vi "LHF.DB.Mongo.Bson.FromVariant.vi"(0 "Variant":variant, 5 "error IO":errorcluster) -> (14 "BsonValue":refnum<k24>, 19 "error IO 2":errorcluster)   [LabVIEW 2013, in "LHF.DB.Mongo.lvclass"]
uses:
  LHF.DB.Mongo.lvclass
  C:/Users/Ricardo/Desktop/Projetos/LabVIEW-MongoDB/src/Driver/MongoDB.Bson.dll
  Driver/MongoDB.Bson.dll
  <vilib>/Utility/VariantDataType/VariantType.lvlib
panel:
  in  "Treatment of Infinity/NaN":T1(ring)
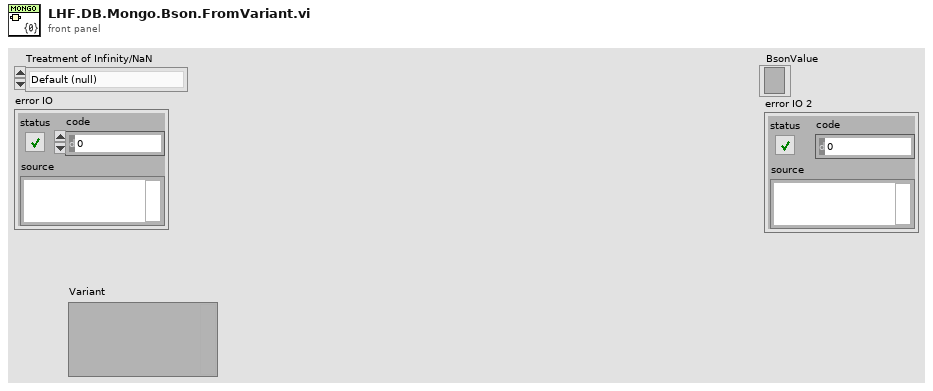
[diagram p1: front panel]
types:
  T1 = enum16{"Default (null)", "Extended", "LabVIEW extensions"}
  T2 = typedef "VariantType.lvlib/Type.ctl" = enum8{"Invalid Type", "Void", "I8", "I16", "I32", "I64", "U8", "U16", "U32", "U64", "Single Float", "Double Float", "Extended Float", "Single Complex", "Double Complex", "Extended Complex", "Enum U8", "Enum U16", "Enum U32", "Enum U64", "Single Float With Unit", "Double Float With Unit", "Extended Float With Unit", "Single Complex with Unit", "Double Complex with Unit", "Extended Complex with Unit", "Boolean", "String", "Path", "Picture", "Tag", "Array", "Cluster", "Variant", "LV Variant", "Waveform", "Timestamp", "Digital Waveform", "Digital Data", "ExpressData", "Refnum", "External Data", "VI", "Poly VI", "LabVIEW Class Instance", "Fixed Point"}
  T3 = typedef "LHF.DB.Mongo.lvclass/LHF.DB.Mongo.Typedef.VariantData.ctl" = cluster{"Type Enum":T2, "Name":string, "Variant":variant}
  T4 = typedef "VariantType.lvlib/RefnumType.ctl" = enum16{"NotARefnum", "UnknownRefnum", "Generic", "Datalog", "ByteStream", "Device", "Occurence", "TCPNetConnection", "Auto", "Menu", "Imaq", "Hardware", "DataSocket", "Visa", "IVI", "UDPNetConnection", "Notifier", "Queue", "Irda", "EventReg", "DotNet", "UserEvent", "Callback", "UNUSED_EMPTY_POSITION", "BlueToothNetConnection", "LVObjApp", "LVObjVI", "LVObjUnknown", "GenericClass", "UserDefinedRefnumTag", "DataValue", "RT FIFO", "TDMS File"}
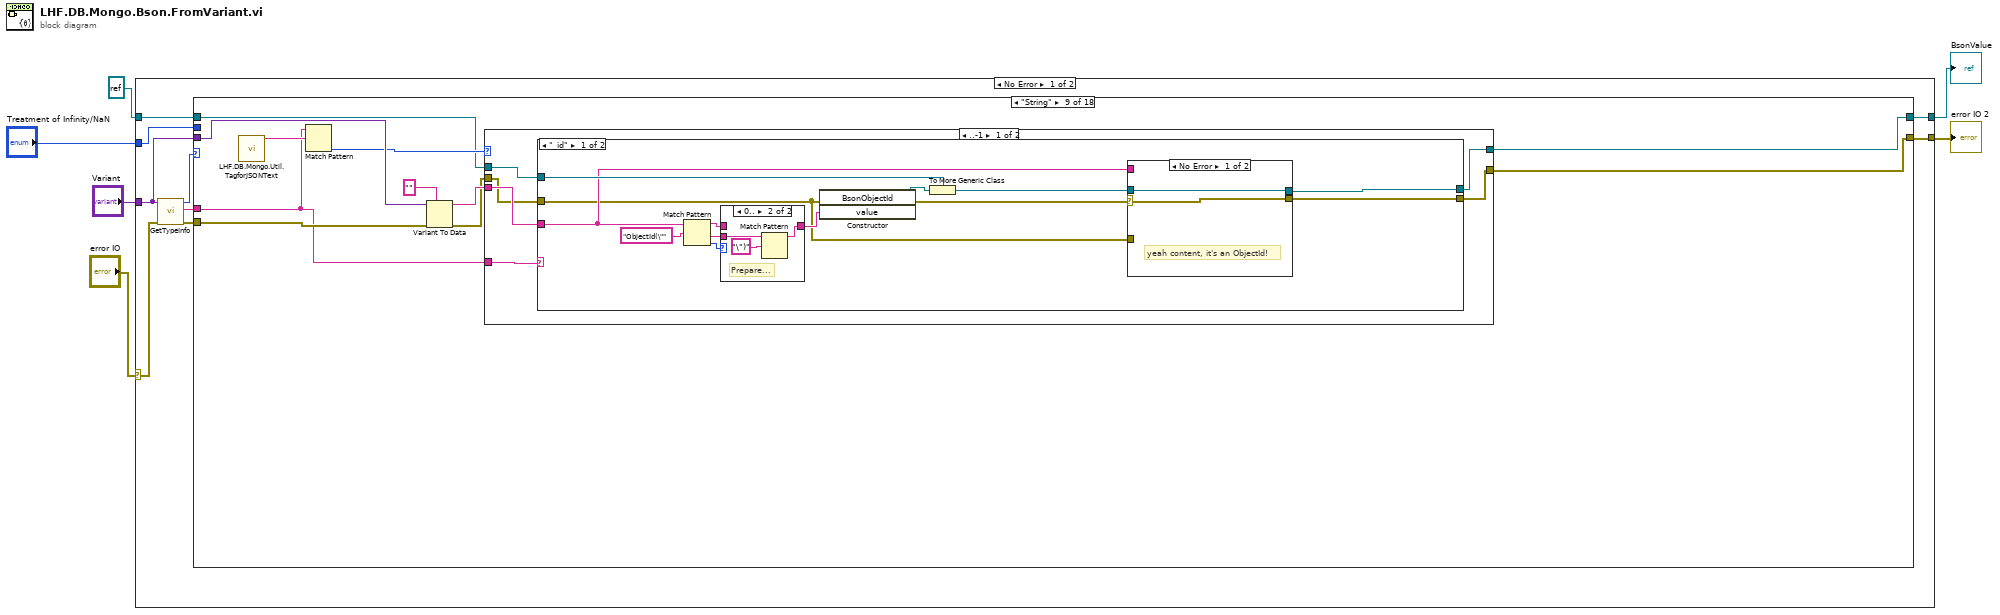
[diagram p0: block diagram]
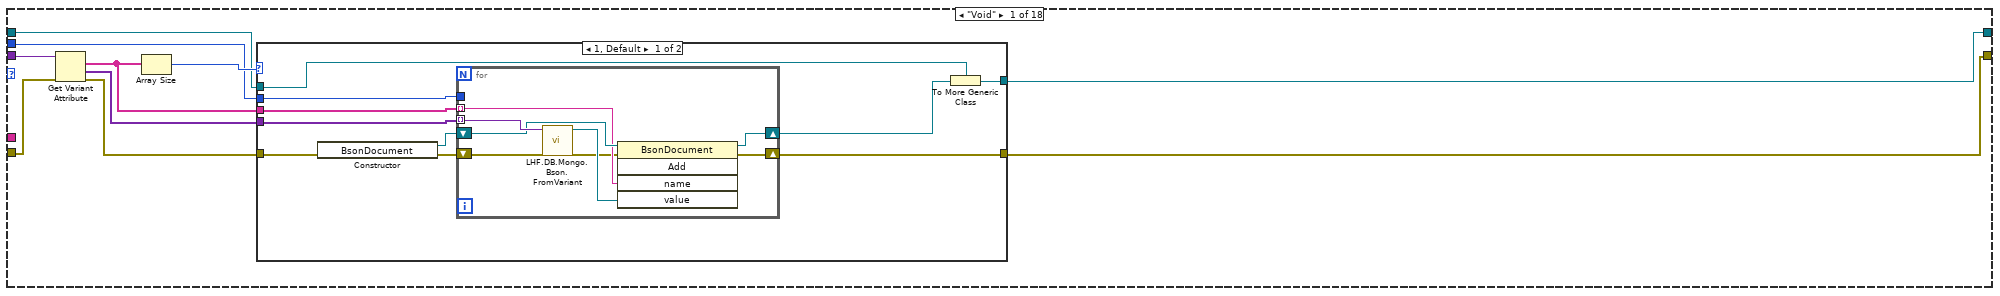
[diagram p2: hidden frame]
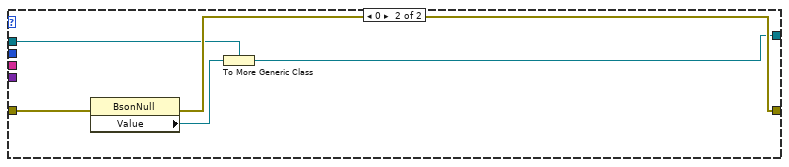
[diagram p3: hidden frame]
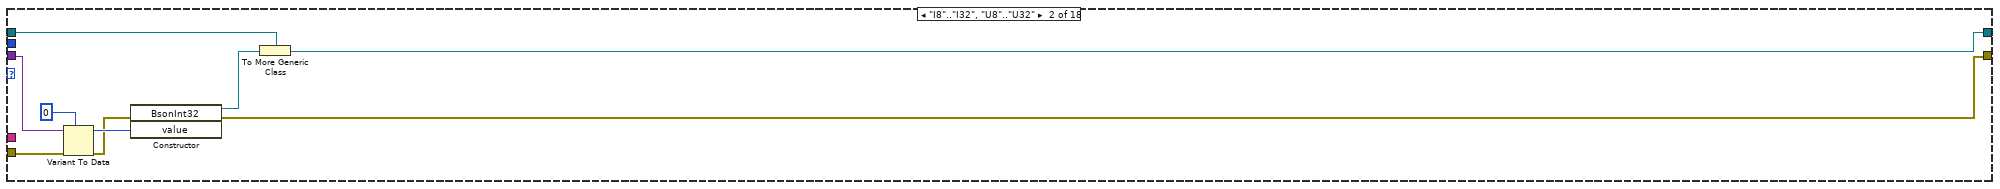
[diagram p4: hidden frame]
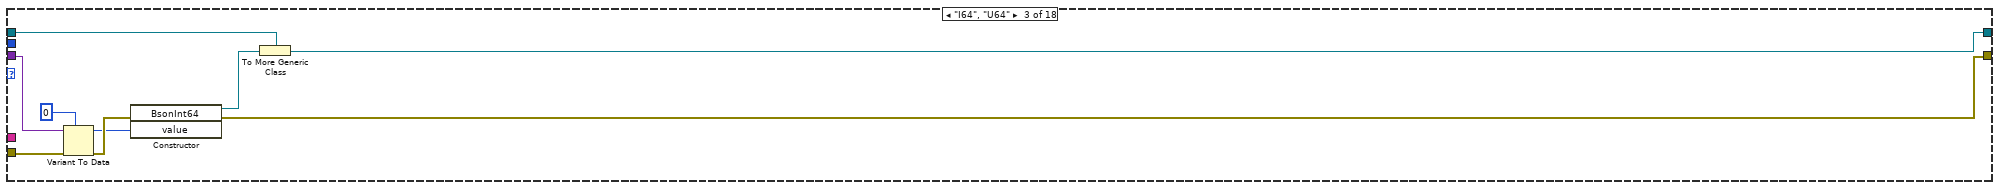
[diagram p5: hidden frame]
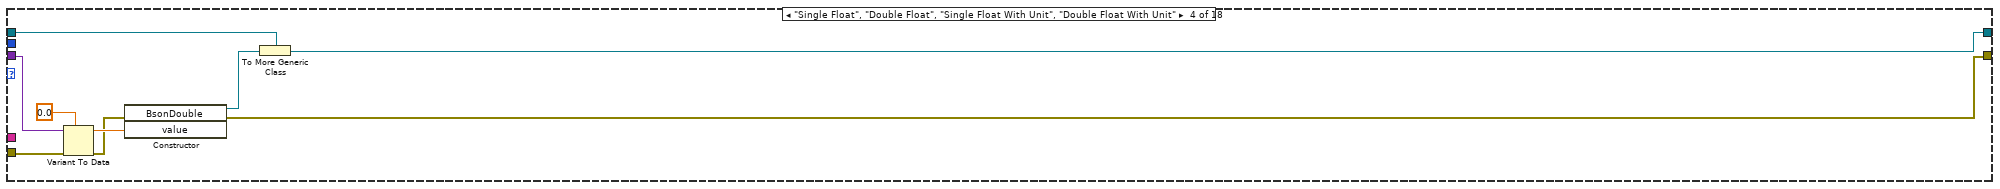
[diagram p6: hidden frame]
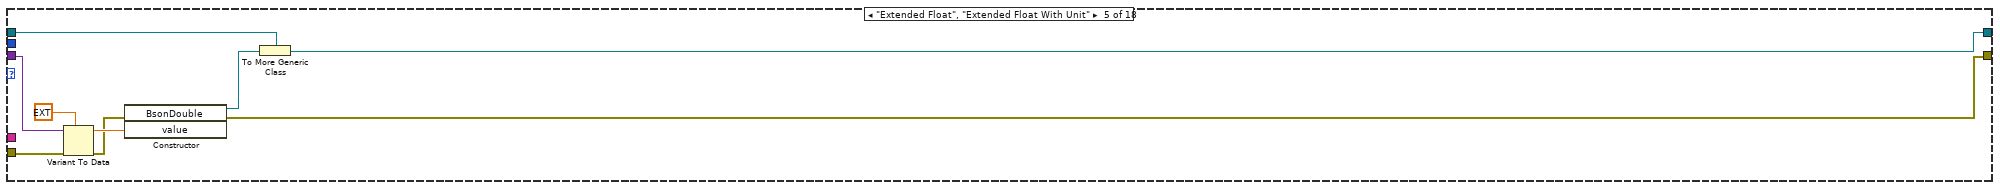
[diagram p7: hidden frame]
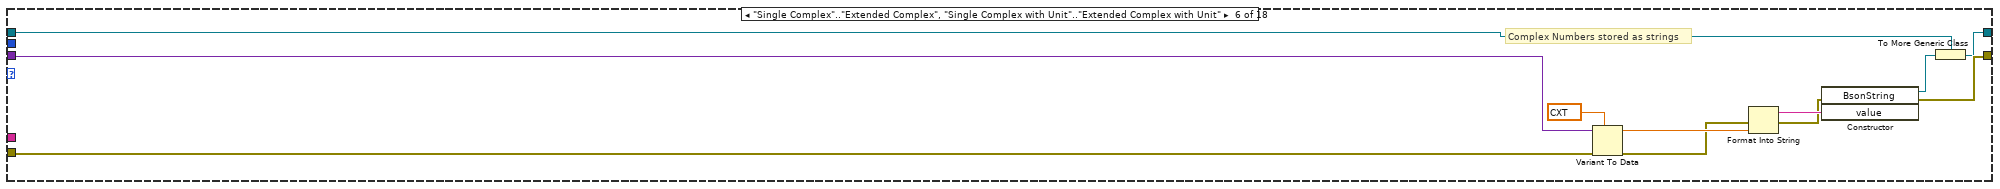
[diagram p8: hidden frame]
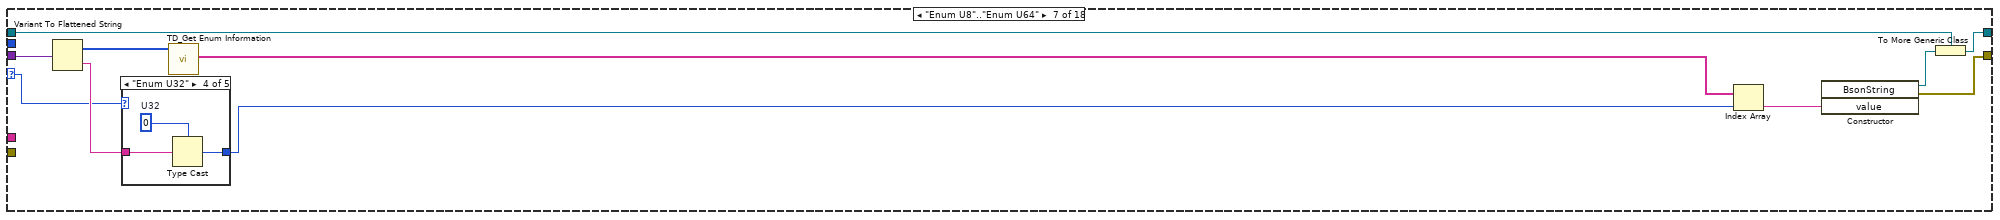
[diagram p9: hidden frame]
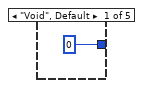
[diagram p10: hidden frame]
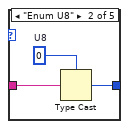
[diagram p11: hidden frame]
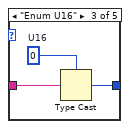
[diagram p12: hidden frame]
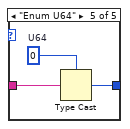
[diagram p13: hidden frame]
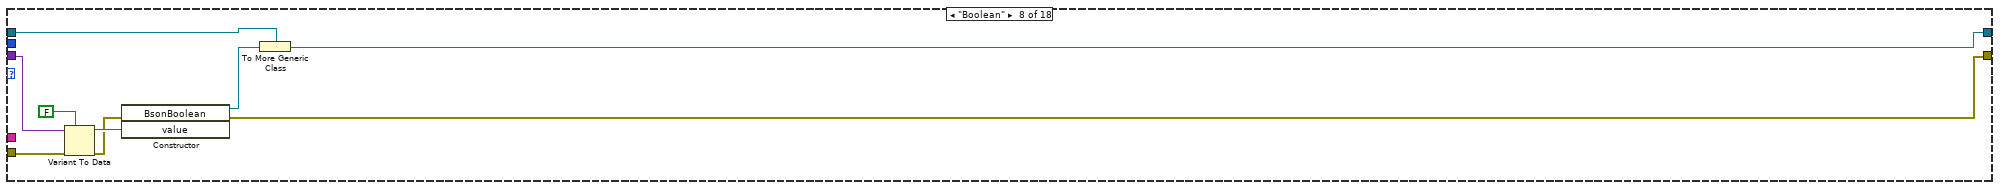
[diagram p14: hidden frame]
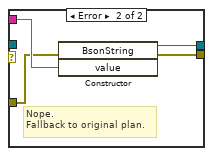
[diagram p15: hidden frame]
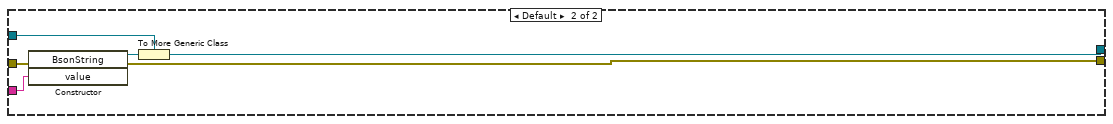
[diagram p17: hidden frame]
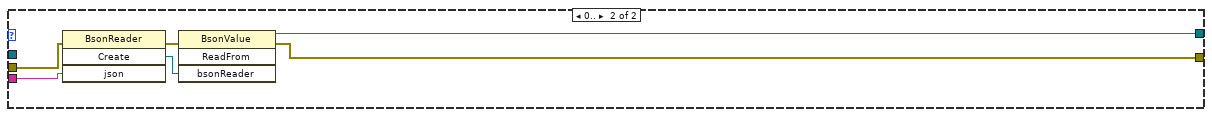
[diagram p18: hidden frame]
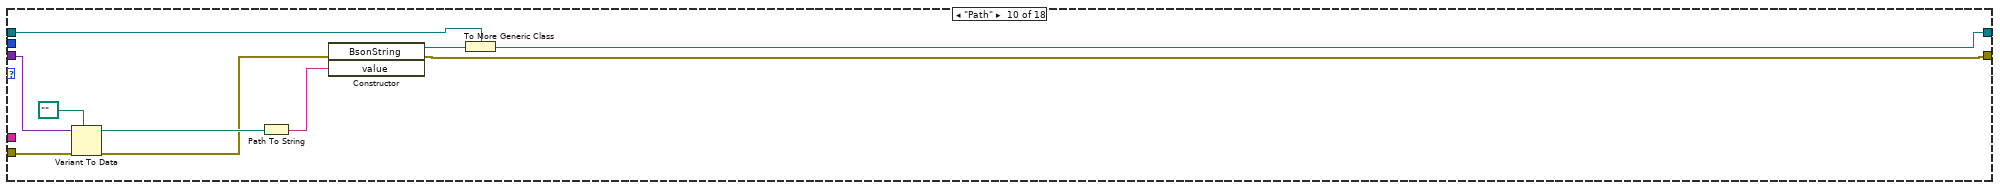
[diagram p19: hidden frame]
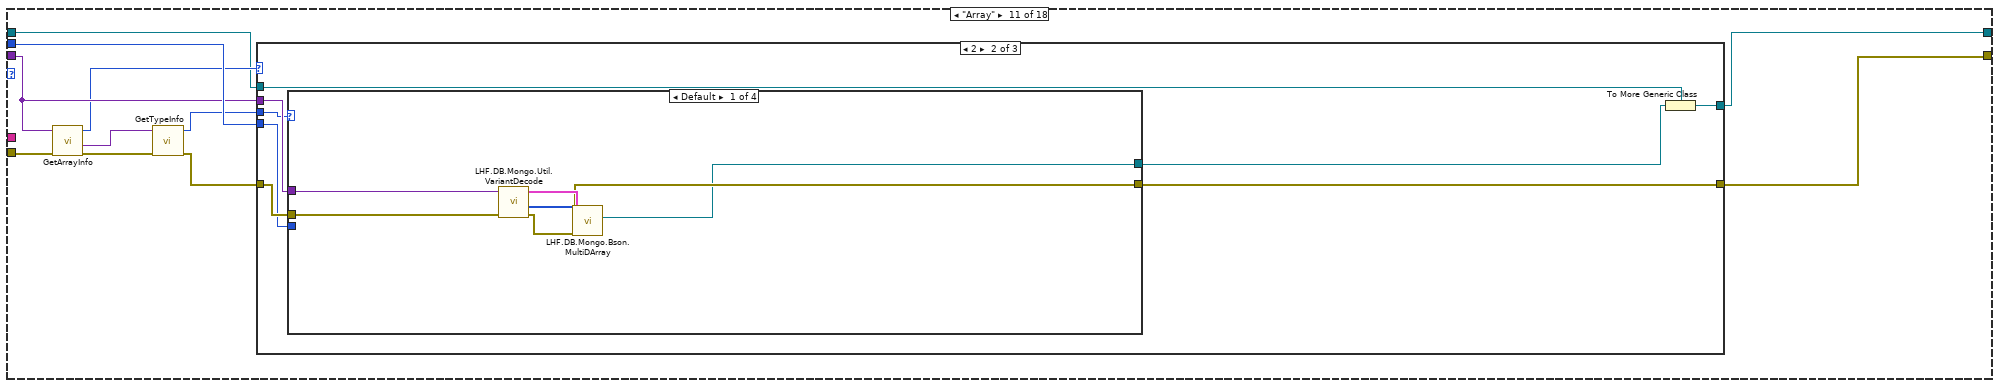
[diagram p20: hidden frame]
diagram:
  n1 = case shown="No Error" "error IO" {
    selector: "error IO" -> [w13 w488]
    tunnel: [w15 w488] -> w1
    tunnel: "Variant" -> [w14 _]
    tunnel: "Treatment of Infinity/NaN" -> [w9 _]
    tunnel: [w8 w487] -> w3
    tunnel: refnum<k24> refnum ("new reference") -> [w7 w487]
    frame No Error {
      n2 = call <vilib>:"GetTypeInfo.vi"("error in (no error)"=w13, "Variant"=w14) -> ("error out"=w12:errorcluster, "Name"=w10:string, "Type Enum"=w11:T2)  [unwired: 5 in, 2 out]
      n3 = case shown="\"String\"" w11 {
        selector: w11 -> [_ _ _ _ _ _ w101 _ _ _ _ _ _ _ _ _ _ _]
        tunnel: w14 -> [w24 w57 w66 w75 w84 w95 w102 w128 w139 w190 w199 w403 w423 w433 w442 w450 w479 w486]
        tunnel: [w25 w52 w63 w68 w79 w88 w98 w122 w135 w184 w201 w405 w419 w428 w437 w444 w471 w482] -> w15
        tunnel: w12 -> [w19 w55 w64 w73 w82 w94 _ w126 w134 w188 w198 w401 w422 w432 w440 w449 w478 w483]
        tunnel: w10 -> [_ _ _ _ _ _ _ _ w129 _ _ _ _ _ _ _ _ _]
        tunnel: w9 -> [w18 _ _ _ _ _ _ _ _ _ w200 w400 _ _ _ _ _ _]
        tunnel: [w16 w49 w58 w67 w76 w85 w96 w120 w131 w181 w191 w396 w416 w425 w435 w443 w469 w480] -> w8
        tunnel: w7 -> [w17 w50 w59 w70 w77 w86 w97 w123 w132 w182 w192 w397 w418 w427 w434 w446 w470 w481]
        frame "Void" {
          n4 = Get Variant Attribute(Variant=w24, error in=w19) -> (names=w22:string[], values=w21:variant[], error out=w20:errorcluster)  [unwired: 2 in, 1 out]
          n5 = Array Size(array=w22) -> (size(s)=w23:i32)
          n6 = case shown="1, Default" w23 {
            tunnel: [w33 w48] -> w25
            tunnel: w22 -> [w34 _]
            tunnel: w21 -> [w35 _]
            tunnel: w20 -> [w26 w47]
            tunnel: w18 -> [w32 _]
            tunnel: w17 -> [w28 w45]
            tunnel: [w29 w44] -> w16
            frame 1, Default {
              n7 = constructor class="BsonDocument"(error in=w26) -> (reference out=w31:refnum<k24>, error out=w27:errorcluster)  [unwired: 2 in, 1 out]
              n8 = for {
                tunnel: w35 -> [w43] mode=indexing
                shift-right: [w36] -> w33
                shift-left: w27 -> [w37]
                tunnel: w34 -> [w40] mode=indexing
                shift-right: [w41] -> w30
                shift-left: w31 -> [w42]
                tunnel: w32 -> [_]
                n9 = call "LHF.DB.Mongo.Bson.FromVariant.vi"("Variant"=w43, "error IO"=w37) -> ("BsonValue"=w39:refnum<k24>, "error IO 2"=w38:errorcluster)  [unwired: 16 in]
                n10 = invoke class="BsonDocument" method="Add"(reference=w42, error in=w38, "name"=w40, "value"=w39) -> (reference out=w41:refnum<k24>, error out=w36:errorcluster)  [unwired: 1 in, 3 out]
              }
              n11 = To More Generic Class(target class=w28, reference=w30) -> (generic class reference=w29:refnum<k24>)
            }
            frame 0 {
              n12 = property class="BsonNull"(error in=w47) -> (error out=w48:errorcluster, "Value"=w46:refnum<k24>)  [unwired: 1 in, 1 out]
              n13 = To More Generic Class(target class=w45, reference=w46) -> (generic class reference=w44:refnum<k24>)
            }
          }
        }
        frame "I8".."I32", "U8".."U32" {
          n14 = Variant To Data(error in=w55, type=0, Variant=w57) -> (data=w54:i32, error out=w53:errorcluster)
          n15 = constructor class="BsonInt32"(error in=w53, "value"=w54) -> (reference out=w51:refnum<k24>, error out=w52:errorcluster)  [unwired: 2 in, 2 out]
          n16 = To More Generic Class(target class=w50, reference=w51) -> (generic class reference=w49:refnum<k24>)
        }
        frame "I64", "U64" {
          n17 = Variant To Data(error in=w64, type=i64 0, Variant=w66) -> (data=w61:i64, error out=w62:errorcluster)
          n18 = constructor class="BsonInt64"(error in=w62, "value"=w61) -> (reference out=w60:refnum<k24>, error out=w63:errorcluster)  [unwired: 2 in, 2 out]
          n19 = To More Generic Class(target class=w59, reference=w60) -> (generic class reference=w58:refnum<k24>)
        }
        frame "Single Float", "Double Float", "Single Float With Unit", "Double Float With Unit" {
          n20 = Variant To Data(error in=w73, type=sgl 0.0, Variant=w75) -> (data=w72:sgl, error out=w69:errorcluster)
          n21 = constructor class="BsonDouble"(error in=w69, "value"=w72) -> (reference out=w71:refnum<k24>, error out=w68:errorcluster)  [unwired: 2 in, 2 out]
          n22 = To More Generic Class(target class=w70, reference=w71) -> (generic class reference=w67:refnum<k24>)
        }
        frame "Extended Float", "Extended Float With Unit" {
          n23 = Variant To Data(error in=w82, type=ext 0.0, Variant=w84) -> (data=w81:ext, error out=w80:errorcluster)
          n24 = constructor class="BsonDouble"(error in=w80, "value"=w81) -> (reference out=w78:refnum<k24>, error out=w79:errorcluster)  [unwired: 2 in, 2 out]
          n25 = To More Generic Class(target class=w77, reference=w78) -> (generic class reference=w76:refnum<k24>)
        }
        frame "Single Complex".."Extended Complex", "Single Complex with Unit".."Extended Complex with Unit" {
          # "Complex Numbers stored as strings"
          n26 = Variant To Data(error in=w94, type=cxt 0.0+0.0i, Variant=w95) -> (data=w92:cxt, error out=w91:errorcluster)
          n27 = Format Into String(error in=w91, w92) -> (resulting string=w90:string, error out=w89:errorcluster)  [unwired: 2 in]
          n28 = constructor class="BsonString"(error in=w89, "value"=w90) -> (reference out=w87:refnum<k24>, error out=w88:errorcluster)  [unwired: 2 in, 2 out]
          n29 = To More Generic Class(target class=w86, reference=w87) -> (generic class reference=w85:refnum<k24>)
        }
        frame "Enum U8".."Enum U64" {
          n30 = Variant To Flattened String(Variant=w102) -> (data string=w105:string, 1:w106:i16[])
          n31 = case shown="\"Enum U32\"" w101 {
            tunnel: w105 -> [_ w110 w113 w116 w119]
            tunnel: [u64 0 ("U8") w108 w111 w114 w117] -> w103
            frame "Void", Default {
            }
            frame "Enum U8" {
              w109 = u8 0  # U8
              n32 = Type Cast(type=w109, x=w110) -> (*(type *) &x=w108:u8)
            }
            frame "Enum U16" {
              w112 = u16 0  # U16
              n33 = Type Cast(type=w112, x=w113) -> (*(type *) &x=w111:u16)
            }
            frame "Enum U32" {
              w115 = u32 0  # U32
              n34 = Type Cast(type=w115, x=w116) -> (*(type *) &x=w114:u32)
            }
            frame "Enum U64" {
              w118 = u64 0  # U64
              n35 = Type Cast(type=w118, x=w119) -> (*(type *) &x=w117:u64)
            }
          }
          n36 = call <vilib>:"TD_Get Enum Information.vi"("Type descriptor"=w106) -> ("Value Names"=w104:string[])  [unwired: 9 in, 1 out]
          n37 = Index Array(array=w104, index=w103) -> (element=w99:string)
          n38 = constructor class="BsonString"("value"=w99) -> (reference out=w100:refnum<k24>, error out=w98:errorcluster)  [unwired: 3 in, 2 out]
          n39 = To More Generic Class(target class=w97, reference=w100) -> (generic class reference=w96:refnum<k24>)
        }
        frame "Boolean" {
          n40 = Variant To Data(error in=w126, type=FALSE, Variant=w128) -> (data=w124:bool, error out=w121:errorcluster)
          n41 = constructor class="BsonBoolean"(error in=w121, "value"=w124) -> (reference out=w125:refnum<k24>, error out=w122:errorcluster)  [unwired: 2 in, 2 out]
          n42 = To More Generic Class(target class=w123, reference=w125) -> (generic class reference=w120:refnum<k24>)
        }
        frame "String" {
          n43 = call "LHF.DB.Mongo.Util.TagforJSONText.vi"() -> ("Tag for JSON text"=w130:string)  [unwired: 11 in]
          n44 = Match Pattern(string=w129, regular expression=w130) -> (offset past match=w133:i32)  [unwired: 1 in, 3 out]
          n45 = Variant To Data(error in=w134, type="", Variant=w139) -> (data=w137:string, error out=w136:errorcluster)
          n46 = case shown="..-1" w133 {
            tunnel: w137 -> [w145 w180]
            tunnel: w136 -> [w141 w177]
            tunnel: [w142 w176] -> w135
            tunnel: [w144 w175] -> w131
            tunnel: w132 -> [w143 _]
            tunnel: w129 -> [w140 _]
            frame ..-1 {
              n47 = case shown="\"_id\"" w140 {
                tunnel: w145 -> [w147 w173]
                tunnel: [w148 w169] -> w144
                tunnel: w143 -> [w152 w172]
                tunnel: [w150 w171] -> w142
                tunnel: w141 -> [w146 w170]
                frame "_id" {
                  n48 = Match Pattern(string=w147, regular expression="ObjectId(\"") -> (before substring=w155:string, after substring=w157:string, offset past match=w156:i32)  [unwired: 1 in, 1 out]
                  n49 = case shown="0.." w156 {
                    tunnel: [w165 w167] -> w154
                    tunnel: w157 -> [_ w166]
                    tunnel: w155 -> [w165 _]
                    frame Default {
                      # "AllReady"
                    }
                    frame 0.. {
                      # "Prepare..."
                      n50 = Match Pattern(string=w166, regular expression="\")") -> (before substring=w167:string)  [unwired: 1 in, 3 out]
                    }
                  }
                  n51 = constructor class="BsonObjectId"(error in=w146, "value"=w154) -> (reference out=w153:refnum<k24>, error out=w151:errorcluster)  [unwired: 2 in, 2 out]
                  n52 = To More Generic Class(target class=w152, reference=w153) -> (generic class reference=w149:refnum<k24>)
                  n53 = case shown="No Error" w151 {
                    selector: w151 -> [w160 _]
                    tunnel: [w160 w162] -> w150
                    tunnel: [w159 w164] -> w148
                    tunnel: w149 -> [w159 _]
                    tunnel: w147 -> [_ w163]
                    tunnel: w146 -> [_ w161]
                    frame No Error {
                      # "yeah content, it's an ObjectId!"
                    }
                    frame Error {
                      # "Nope.\nFallback to original plan."
                      n54 = constructor class="BsonString"(error in=w161, "value"=w163) -> (reference out=w164:refnum<k24>, error out=w162:errorcluster)  [unwired: 2 in, 2 out]
                    }
                  }
                }
                frame Default {
                  n55 = constructor class="BsonString"(error in=w170, "value"=w173) -> (reference out=w174:refnum<k24>, error out=w171:errorcluster)  [unwired: 2 in, 2 out]
                  n56 = To More Generic Class(target class=w172, reference=w174) -> (generic class reference=w169:refnum<k24>)
                }
              }
            }
            frame 0.. {
              n57 = invoke class="BsonReader" method="Create"(error in=w177, "json"=w180) -> (error out=w178:errorcluster, "Create"=w179:refnum<k24>)  [unwired: 2 in, 2 out]
              n58 = invoke class="BsonValue" method="ReadFrom"(error in=w178, "bsonReader"=w179) -> (reference out=w175:refnum<k24>, error out=w176:errorcluster)  [unwired: 2 in, 2 out]
            }
          }
        }
        frame "Path" {
          n59 = Variant To Data(error in=w188, type=path "", Variant=w190) -> (data=w187:path, error out=w185:errorcluster)
          n60 = Path To String(path=w187) -> (string=w186:string)
          n61 = constructor class="BsonString"(error in=w185, "value"=w186) -> (reference out=w183:refnum<k24>, error out=w184:errorcluster)  [unwired: 2 in, 2 out]
          n62 = To More Generic Class(target class=w182, reference=w183) -> (generic class reference=w181:refnum<k24>)
        }
        frame "Array" {
          n63 = call <vilib>:"GetArrayInfo.vi"("error in (no error)"=w198, "Variant"=w199) -> ("error out"=w196:errorcluster, "ArrayElement"=w195:variant, "NDims"=w197:i32)  [unwired: 6 in, 1 out]
          n64 = call <vilib>:"GetTypeInfo.vi"("error in (no error)"=w196, "Variant"=w195) -> ("error out"=w194:errorcluster, "Type Enum"=w193:T2)  [unwired: 5 in, 3 out]
          n65 = case shown="2" w197 {
            tunnel: [w210 w309 w395] -> w201
            tunnel: w200 -> [w209 w307 _]
            tunnel: w199 -> [w211 w310 w391]
            tunnel: w194 -> [w207 w308 w390]
            tunnel: w193 -> [w208 w306 _]
            tunnel: w192 -> [w203 w303 w387]
            tunnel: [w202 w304 w388] -> w191
            frame 1 {
              n66 = constructor class="BsonArray"(error in=w207) -> (reference out=w205:refnum<k24>, error out=w206:errorcluster)  [unwired: 2 in, 1 out]
              n67 = case shown="Default" w208 {
                tunnel: w211 -> [w215 w234 w249 w264 w279 w295]
                tunnel: [w216 w227 w242 w258 w274 w287] -> w210
                tunnel: w206 -> [w213 w232 w247 w262 w275 w291]
                tunnel: w209 -> [w219 _ _ _ _ w290]
                tunnel: w205 -> [w218 w230 w246 w260 w273 w289]
                tunnel: [w217 w228 w243 w259 w272 w288] -> w204
                frame Default {
                  n68 = call <userlib>:"Array to Array of VData__ogtk.vi"("error in (no error)"=w213, "MultiD Array"=w215) -> ("error out"=w212:errorcluster, "1D Array of Variants"=w214:variant[])  [unwired: 8 in]
                  n69 = for {
                    shift-right: [w222] -> w216
                    shift-left: w212 -> [w226]
                    tunnel: w219 -> [_]
                    shift-right: [w223] -> w217
                    shift-left: w218 -> [w224]
                    tunnel: w214 -> [w220] mode=indexing
                    n70 = call "LHF.DB.Mongo.Bson.FromVariant.vi"("Variant"=w220, "error IO"=w226) -> ("BsonValue"=w225:refnum<k24>, "error IO 2"=w221:errorcluster)  [unwired: 16 in]
                    n71 = invoke class="BsonArray" method="Add"(reference=w224, error in=w221, "value"=w225) -> (reference out=w223:refnum<k24>, error out=w222:errorcluster)  [unwired: 1 in, 2 out]
                  }
                }
                frame "Single Float".."Extended Float" {
                  n72 = Variant To Data(error in=w232, type=sgl[] [], Variant=w234) -> (data=w229:sgl[], error out=w231:errorcluster)
                  n73 = for {
                    shift-right: [w239] -> w228
                    shift-left: w230 -> [w241]
                    shift-right: [w238] -> w227
                    shift-left: w231 -> [w237]
                    tunnel: w229 -> [w235] mode=indexing
                    n74 = constructor class="BsonDouble"(error in=w237, "value"=w235) -> (reference out=w240:refnum<k24>, error out=w236:errorcluster)  [unwired: 2 in, 2 out]
                    n75 = invoke class="BsonArray" method="Add"(reference=w241, error in=w236, "value"=w240) -> (reference out=w239:refnum<k24>, error out=w238:errorcluster)  [unwired: 1 in, 2 out]
                  }
                }
                frame "I8".."I32", "U8".."U32" {
                  n76 = Variant To Data(error in=w247, type=i32[] [], Variant=w249) -> (data=w244:i32[], error out=w245:errorcluster)
                  n77 = for {
                    shift-right: [w254] -> w243
                    shift-left: w246 -> [w256]
                    shift-right: [w253] -> w242
                    shift-left: w245 -> [w252]
                    tunnel: w244 -> [w250] mode=indexing
                    n78 = constructor class="BsonInt32"(error in=w252, "value"=w250) -> (reference out=w255:refnum<k24>, error out=w251:errorcluster)  [unwired: 2 in, 2 out]
                    n79 = invoke class="BsonArray" method="Add"(reference=w256, error in=w251, "value"=w255) -> (reference out=w254:refnum<k24>, error out=w253:errorcluster)  [unwired: 1 in, 2 out]
                  }
                }
                frame "I64", "U64" {
                  n80 = Variant To Data(error in=w262, type=i64[] [], Variant=w264) -> (data=w257:i64[], error out=w261:errorcluster)
                  n81 = for {
                    shift-right: [w269] -> w259
                    shift-left: w260 -> [w271]
                    shift-right: [w268] -> w258
                    shift-left: w261 -> [w267]
                    tunnel: w257 -> [w265] mode=indexing
                    n82 = constructor class="BsonInt64"(error in=w267, "value"=w265) -> (reference out=w270:refnum<k24>, error out=w266:errorcluster)  [unwired: 2 in, 2 out]
                    n83 = invoke class="BsonArray" method="Add"(reference=w271, error in=w266, "value"=w270) -> (reference out=w269:refnum<k24>, error out=w268:errorcluster)  [unwired: 1 in, 2 out]
                  }
                }
                frame "Timestamp" {
                  n84 = Variant To Data(error in=w275, type=timestamp[] [], Variant=w279) -> (data=w277:timestamp[], error out=w276:errorcluster)
                  n85 = for {
                    tunnel: w277 -> [w286] mode=indexing
                    shift-right: [w280] -> w274
                    shift-left: w276 -> [w285]
                    shift-right: [w282] -> w272
                    shift-left: w273 -> [w283]
                    n86 = call "LHF.DB.Mongo.Bson.Timestamp.vi"("t0"=w286, "error in (no error)"=w285) -> ("BsonString"=w284:refnum<k24>, "error out"=w281:errorcluster)  [unwired: 16 in]
                    n87 = invoke class="BsonArray" method="Add"(reference=w283, error in=w281, "value"=w284) -> (reference out=w282:refnum<k24>, error out=w280:errorcluster)  [unwired: 1 in, 2 out]
                  }
                }
                frame "Waveform" {
                  n88 = Variant To Data(error in=w291, type=waveform(dbl)[] [], Variant=w295) -> (data=w293:waveform(dbl)[], error out=w292:errorcluster)
                  n89 = for {
                    tunnel: w293 -> [w301] mode=indexing
                    shift-right: [w297] -> w287
                    shift-left: w292 -> [w302]
                    tunnel: w290 -> [_]
                    shift-right: [w298] -> w288
                    shift-left: w289 -> [w299]
                    n90 = call "LHF.DB.Mongo.Bson.Waveform.vi"("waveform"=w301, "error in (no error)"=w302) -> ("BsonDocument"=w300:refnum<k24>, "error out"=w296:errorcluster)  [unwired: 16 in]
                    n91 = invoke class="BsonArray" method="Add"(reference=w299, error in=w296, "value"=w300) -> (reference out=w298:refnum<k24>, error out=w297:errorcluster)  [unwired: 1 in, 2 out]
                  }
                }
              }
              n92 = To More Generic Class(target class=w203, reference=w204) -> (generic class reference=w202:refnum<k24>)
            }
            frame 2 {
              n93 = case shown="Default" w306 {
                tunnel: w310 -> [w314 w325 w347 w371]
                tunnel: [w312 w322 w345 w364] -> w309
                tunnel: w308 -> [w313 w324 w348 w367]
                tunnel: w307 -> [_ _ _ _]
                tunnel: [w311 w323 w346 w365] -> w305
                frame Default {
                  n94 = call "LHF.DB.Mongo.Util.VariantDecode.vi"("error in (no error)"=w313, "variant"=w314) -> ("error out"=w317:errorcluster, "Array Dimensions (Reversed)"=w315:i32[], "Variant Data"=w316:T3[])  [unwired: 7 in]
                  n95 = call "LHF.DB.Mongo.Bson.MultiDArray.vi"("error in (no error)"=w317, "Array Dimensions"=w315, "Variant Data"=w316) -> ("error out"=w312:errorcluster, "BsonArray"=w311:refnum<k24>)  [unwired: 6 in, 1 out]
                }
                frame "Single Float".."Extended Float" {
                  n96 = constructor class="BsonArray"() -> (reference out=w319:refnum<k24>)  [unwired: 3 in, 2 out]
                  n97 = Variant To Data(error in=w324, type=dbl[][] [], Variant=w325) -> (data=w321:dbl[][], error out=w320:errorcluster)
                  n98 = for {
                    tunnel: w321 -> [w333] mode=indexing
                    tunnel: w320 -> [w332]
                    shift-right: [w329] -> w322
                    shift-left: _ -> [_]
                    shift-right: [w326] -> w323
                    shift-left: w319 -> [w327]
                    n99 = constructor class="BsonArray"() -> (reference out=w331:refnum<k24>)  [unwired: 3 in, 2 out]
                    n100 = for {
                      tunnel: w333 -> [w338] mode=indexing
                      shift-right: [w336] -> w330
                      shift-left: w332 -> [w334]
                      shift-right: [w335] -> w328
                      shift-left: w331 -> [w337]
                      n101 = constructor class="BsonDouble"(error in=w334, "value"=w338) -> (reference out=w340:refnum<k24>, error out=w339:errorcluster)  [unwired: 2 in, 2 out]
                      n102 = invoke class="BsonArray" method="Add"(reference=w337, error in=w339, "value"=w340) -> (reference out=w335:refnum<k24>, error out=w336:errorcluster)  [unwired: 1 in, 2 out]
                    }
                    n103 = invoke class="BsonArray" method="Add"(reference=w327, error in=w330, "value"=w328) -> (reference out=w326:refnum<k24>, error out=w329:errorcluster)  [unwired: 1 in, 2 out]
                  }
                }
                frame "I8".."I32", "U8".."U32" {
                  n104 = Variant To Data(error in=w348, type=i32[][] [], Variant=w347) -> (data=w344:i32[][], error out=w343:errorcluster)
                  n105 = constructor class="BsonArray"() -> (reference out=w342:refnum<k24>)  [unwired: 3 in, 2 out]
                  n106 = for {
                    tunnel: w344 -> [w356] mode=indexing
                    tunnel: w343 -> [w355]
                    shift-right: [w352] -> w345
                    shift-left: _ -> [_]
                    shift-right: [w349] -> w346
                    shift-left: w342 -> [w350]
                    n107 = constructor class="BsonArray"() -> (reference out=w354:refnum<k24>)  [unwired: 3 in, 2 out]
                    n108 = for {
                      tunnel: w356 -> [w361] mode=indexing
                      shift-right: [w359] -> w353
                      shift-left: w355 -> [w357]
                      shift-right: [w358] -> w351
                      shift-left: w354 -> [w360]
                      n109 = constructor class="BsonInt32"(error in=w357, "value"=w361) -> (reference out=w363:refnum<k24>, error out=w362:errorcluster)  [unwired: 2 in, 2 out]
                      n110 = invoke class="BsonArray" method="Add"(reference=w360, error in=w362, "value"=w363) -> (reference out=w358:refnum<k24>, error out=w359:errorcluster)  [unwired: 1 in, 2 out]
                    }
                    n111 = invoke class="BsonArray" method="Add"(reference=w350, error in=w353, "value"=w351) -> (reference out=w349:refnum<k24>, error out=w352:errorcluster)  [unwired: 1 in, 2 out]
                  }
                }
                frame "I64", "U64" {
                  n112 = Variant To Data(error in=w367, type=i64[][] [], Variant=w371) -> (data=w369:i64[][], error out=w368:errorcluster)
                  n113 = constructor class="BsonArray"() -> (reference out=w366:refnum<k24>)  [unwired: 3 in, 2 out]
                  n114 = for {
                    tunnel: w369 -> [w379] mode=indexing
                    tunnel: w368 -> [w378]
                    shift-right: [w375] -> w364
                    shift-left: _ -> [_]
                    shift-right: [w372] -> w365
                    shift-left: w366 -> [w373]
                    n115 = constructor class="BsonArray"() -> (reference out=w377:refnum<k24>)  [unwired: 3 in, 2 out]
                    n116 = for {
                      tunnel: w379 -> [w384] mode=indexing
                      shift-right: [w382] -> w376
                      shift-left: w378 -> [w380]
                      shift-right: [w381] -> w374
                      shift-left: w377 -> [w383]
                      n117 = constructor class="BsonInt64"(error in=w380, "value"=w384) -> (reference out=w386:refnum<k24>, error out=w385:errorcluster)  [unwired: 2 in, 2 out]
                      n118 = invoke class="BsonArray" method="Add"(reference=w383, error in=w385, "value"=w386) -> (reference out=w381:refnum<k24>, error out=w382:errorcluster)  [unwired: 1 in, 2 out]
                    }
                    n119 = invoke class="BsonArray" method="Add"(reference=w373, error in=w376, "value"=w374) -> (reference out=w372:refnum<k24>, error out=w375:errorcluster)  [unwired: 1 in, 2 out]
                  }
                }
              }
              n120 = To More Generic Class(target class=w303, reference=w305) -> (generic class reference=w304:refnum<k24>)
            }
            frame Default {
              n121 = call "LHF.DB.Mongo.Util.VariantDecode.vi"("error in (no error)"=w390, "variant"=w391) -> ("error out"=w394:errorcluster, "Array Dimensions (Reversed)"=w392:i32[], "Variant Data"=w393:T3[])  [unwired: 7 in]
              n122 = call "LHF.DB.Mongo.Bson.MultiDArray.vi"("error in (no error)"=w394, "Array Dimensions"=w392, "Variant Data"=w393) -> ("error out"=w395:errorcluster, "BsonArray"=w389:refnum<k24>)  [unwired: 6 in, 1 out]
              n123 = To More Generic Class(target class=w387, reference=w389) -> (generic class reference=w388:refnum<k24>)
            }
          }
        }
        frame "Cluster" {
          (unwired) refnum<k24> refnum ("new reference")
          n124 = constructor class="BsonDocument"() -> (reference out=w399:refnum<k24>)  [unwired: 3 in, 2 out]
          n125 = call "LHF.DB.Mongo.Util.VariantDecode.vi"("error in (no error)"=w401, "variant"=w403) -> ("error out"=w402:errorcluster, "Variant Data"=w404:T3[])  [unwired: 7 in, 1 out]
          n126 = for {
            shift-right: [w409] -> w398
            shift-left: w399 -> [w408]
            shift-right: [w407] -> w405
            shift-left: w402 -> [w410]
            tunnel: w404 -> [w415] mode=indexing
            tunnel: w400 -> [_]
            n127 = call "LHF.DB.Mongo.Util.HandleJSONTextTag.vi"("Variant Data"=w415) -> ("Variant Data (tag stripped)"=w414:T3)  [unwired: 9 in, 1 out]
            n128 = Unbundle By Name(w414) -> ("Name"=w413:string, "Variant"=w412:variant)
            n129 = call "LHF.DB.Mongo.Bson.FromVariant.vi"("Variant"=w412, "error IO"=w410) -> ("BsonValue"=w411:refnum<k24>, "error IO 2"=w406:errorcluster)  [unwired: 16 in]
            n130 = invoke class="BsonDocument" method="Add"(reference=w408, error in=w406, "name"=w413, "value"=w411) -> (error out=w407:errorcluster, "Add"=w409:refnum<k24>)  [unwired: 1 in, 3 out]
          }
          n131 = To More Generic Class(target class=w397, reference=w398) -> (generic class reference=w396:refnum<k24>)
        }
        frame "Variant", "LV Variant" {
          n132 = Variant To Data(error in=w422, type=variant, Variant=w423) -> (data=w421:variant, error out=w420:errorcluster)
          n133 = call "LHF.DB.Mongo.Bson.FromVariant.vi"("Variant"=w421, "error IO"=w420) -> ("BsonValue"=w417:refnum<k24>, "error IO 2"=w419:errorcluster)  [unwired: 16 in]
          n134 = To More Generic Class(target class=w418, reference=w417) -> (generic class reference=w416:refnum<k24>)
        }
        frame "Waveform" {
          n135 = Variant To Data(error in=w432, type=waveform(dbl) {"t0"=timestamp(0 s since 1904-01-01), "dt"=1.0, "Y"=[]} ("waveform"), Variant=w433) -> (data=w430:waveform(dbl), error out=w426:errorcluster)
          n136 = call "LHF.DB.Mongo.Bson.Waveform.vi"("waveform"=w430, "error in (no error)"=w426) -> ("BsonDocument"=w429:refnum<k24>, "error out"=w428:errorcluster)  [unwired: 16 in]
          n137 = To More Generic Class(target class=w427, reference=w429) -> (generic class reference=w425:refnum<k24>)
        }
        frame "Timestamp" {
          n138 = Variant To Data(error in=w440, type=timestamp(0 s since 1904-01-01), Variant=w442) -> (data=w439:timestamp, error out=w438:errorcluster)
          n139 = call "LHF.DB.Mongo.Bson.Timestamp.vi"("t0"=w439, "error in (no error)"=w438) -> ("BsonString"=w436:refnum<k24>, "error out"=w437:errorcluster)  [unwired: 16 in]
          n140 = To More Generic Class(target class=w434, reference=w436) -> (generic class reference=w435:refnum<k24>)
        }
        frame "Refnum" {
          n141 = call <vilib>:"GetRefnumInfo.vi"("error in (no error)"=w449, "Variant"=w450) -> ("error out"=w452:errorcluster, "ReferenceType"=w451:T4)  [unwired: 6 in, 2 out]
          n142 = case shown="Default" w451 {
            selector: w451 -> [w455 _ _]
            tunnel: [w454 w458 w462] -> w447
            tunnel: w452 -> [w456 w460 w464]
            tunnel: [w453 w457 w463] -> w445
            tunnel: w450 -> [_ w461 w467]
            frame "NotARefnum", "UnknownRefnum" {
              n143 = call <userlib>:"Get Strings from Enum__ogtk.vi"("error in (no error)"=w456, "Enum"=w455) -> ("error out"=w453:errorcluster, "String Value"=w454:string)  [unwired: 6 in, 2 out]
            }
            frame "Visa", "IVI", "UserDefinedRefnumTag" {
              n144 = Variant To Data(error in=w460, type="", Variant=w461) -> (data=w458:string, error out=w457:errorcluster)
            }
            frame Default {
              n145 = Variant To Flattened String(Variant=w467) -> (data string=w466:string)  [unwired: 1 out]
              n146 = Type Cast(type=0, x=w466) -> (*(type *) &x=w465:i32)
              n147 = Format Into String(error in=w464, w465) -> (resulting string=w462:string, error out=w463:errorcluster)  [unwired: 2 in]
            }
          }
          n148 = constructor class="BsonString"(error in=w445, "value"=w447) -> (reference out=w448:refnum<k24>, error out=w444:errorcluster)  [unwired: 2 in, 2 out]
          n149 = To More Generic Class(target class=w446, reference=w448) -> (generic class reference=w443:refnum<k24>)
        }
        frame "LabVIEW Class Instance" {
          n150 = Variant To Data(error in=w478, type=refnum<class> refnum ("LabVIEW Object"), Variant=w479) -> (data=w476:refnum<class>, error out=w472:errorcluster)
          n151 = Flatten To String(anything=w476, error in (no error)=w472) -> (data string=w474:string, error out=w473:errorcluster)  [unwired: 2 in, 1 out]
          n152 = constructor class="BsonString"(error in=w473, "value"=w474) -> (reference out=w475:refnum<k24>, error out=w471:errorcluster)  [unwired: 2 in, 2 out]
          n153 = To More Generic Class(target class=w470, reference=w475) -> (generic class reference=w469:refnum<k24>)
        }
        frame Default {
          n154 = Variant To Flattened String(Variant=w486) -> (data string=w484:string)  [unwired: 1 out]
          n155 = constructor class="BsonString"(error in=w483, "value"=w484) -> (reference out=w485:refnum<k24>, error out=w482:errorcluster)  [unwired: 2 in, 2 out]
          n156 = To More Generic Class(target class=w481, reference=w485) -> (generic class reference=w480:refnum<k24>)
        }
      }
    }
    frame Error {
    }
  }
  "BsonValue" <- w3
  "error IO 2" <- w1
